vi "DFD Convert FXP to Integer.vi"   [LabVIEW 2017, in "NI_DigFilterLicensed.lvlib"]
doc: "Converts fixed-point numbers to integers. You must manually select the polymorphic instance you want to use."
uses:
  <vilib>/addons/Digital Filter Design/NI_DigFilterLicensed.lvlib
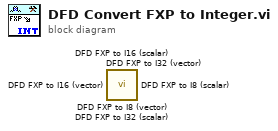
[diagram p0: block diagram]
diagram:
  n1 = call <vilib>:"DFD FXP to I8 (vector).vi"() -> ()  [unwired: 10 in, 2 out]
  n2 = call <vilib>:"DFD FXP to I32 (vector).vi"() -> ()  [unwired: 10 in, 2 out]
  n3 = call <vilib>:"DFD FXP to I16 (vector).vi"() -> ()  [unwired: 10 in, 2 out]
  n4 = call <vilib>:"DFD FXP to I8 (scalar).vi"() -> ()  [unwired: 10 in, 2 out]
  n5 = call <vilib>:"DFD FXP to I32 (scalar).vi"() -> ()  [unwired: 10 in, 2 out]
  n6 = call <vilib>:"DFD FXP to I16 (scalar).vi"() -> ()  [unwired: 10 in, 2 out]
